vi "Read_DR_DATA.vi"(10 "文件路径":path caption="文件路径 （空时为对话框）") -> (0 "标尺号":i32[](array[numeric]), 1 "时间步长":dbl, 2 "P2数据":dbl[][](array[numeric]), 3 "通量数据":dbl[][](array[numeric]), 4 "曲线数据":dbl[][](array[numeric]), 5 "读取正确?":bool, 6 "曲线名称":string[](array[string]), 8 "数据采集起止时间":string, 11 "filepath":path caption="数据文件路径和名称")   [LabVIEW 2020]
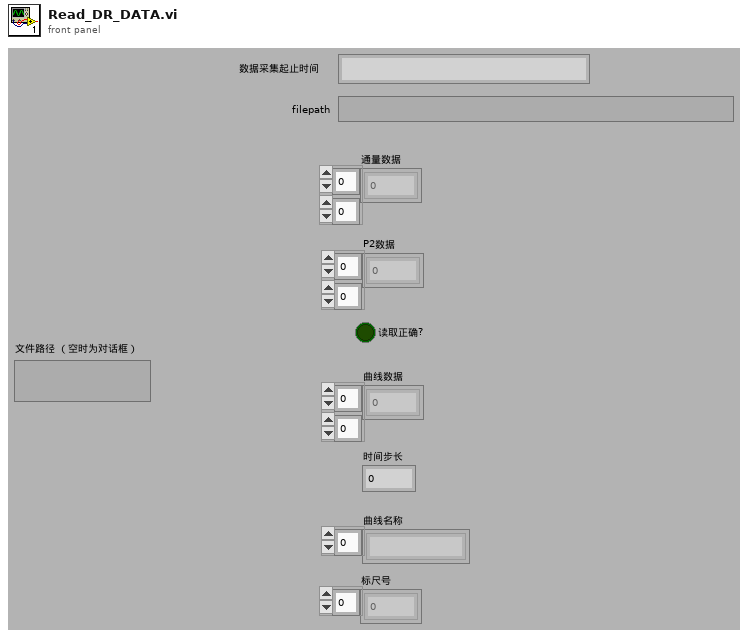
[diagram p1: front panel]
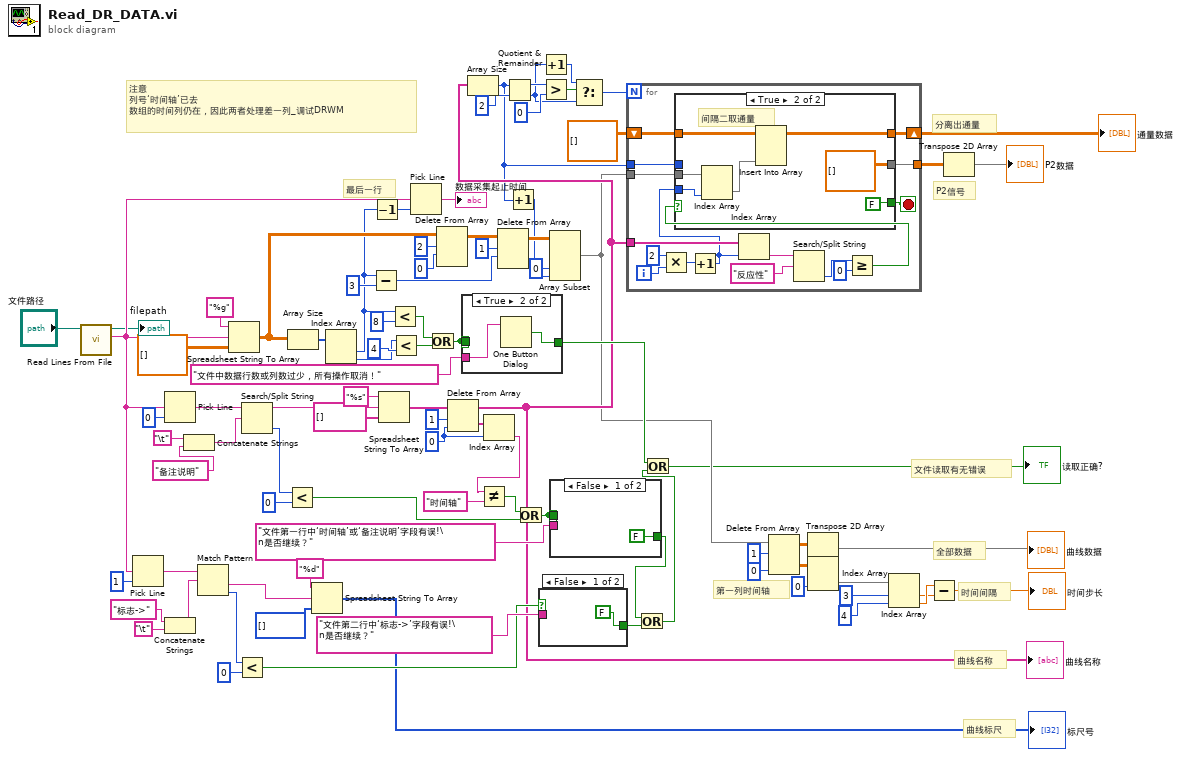
[diagram p0: block diagram]
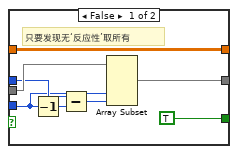
[diagram p2: hidden frame]
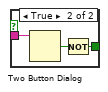
[diagram p3: hidden frame]
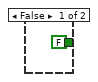
[diagram p4: hidden frame]
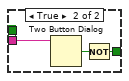
[diagram p5: hidden frame]
diagram:
  w49 = 0 ("索引")
  # "文件读取有无错误"
  # "P2信号"
  # "曲线标尺"
  # "曲线名称"
  # "时间间隔"
  # "全部数据"
  # "分离出通量"
  # "注意\n列号‘时间轴’已去\n数组的时间列仍在，因此两者处理差一列_调试DRWM"
  # "第一列时间轴"
  # "最后一行"
  n1 = call <vilib>:"Read Lines From File.vi"("file path (dialog if empty)"="文件路径") -> ("new file path (Not A Path if cancelled)"=→"filepath":path, "line string"=w39:string)  [unwired: 5 in, 2 out]
  n2 = Pick Line(multi-line string=w39, line index=1 ("行索引")) -> (output string=w66:string)  [unwired: 1 in]
  n3 = Pick Line(multi-line string=w39, line index=0 ("行索引")) -> (output string=w84:string)  [unwired: 1 in]
  n4 = Concatenate Strings("标志->" ("搜索字符串/字符(-)"), "\t") -> (w63:string)
  n5 = Concatenate Strings("\t", "备注说明" ("搜索字符串/字符(-)")) -> (w42:string)
  n6 = Match Pattern(string=w66, regular expression=w63) -> (after substring=w60:string, offset past match=w54:i32)  [unwired: 1 in, 2 out]
  n7 = Spreadsheet String To Array ("电子表格字符串至数组转换")(format string="%g" ("format (%.3f)"), spreadsheet string=w39, array type (2D Dbl)=dbl[][] [] ("type (empty)")) -> (array=w44:dbl[][])  [unwired: 1 in]
  n8 = Less?(x=w54, y=0) -> (x < y?=w53:bool)
  n9 = Search/Split String(string=w84, search string/char (-)=w42) -> (substring before match=w83:string, offset of match=w82:i32)  [unwired: 1 in, 1 out]
  n10 = Less?(x=w82, y=0) -> (x < y?=w79:bool)
  n11 = Array Size(array=w44) -> (size(s)=w90:i32[])
  n12 = Spreadsheet String To Array ("电子表格字符串至数组转换")(format string="%d" ("format (%.3f)"), spreadsheet string=w60, array type (2D Dbl)=i32[] [] ("添加的数组")) -> (array=→"标尺号":i32[])  [unwired: 1 in]
  n13 = Index Array(array=w90) -> (element #1=w12:i32, element #2=w73:i32)  [unwired: 2 in]
  n14 = Subtract(x=w12, y=3) -> (x-y=w38:i32)
  n15 = Decrement(x=w12) -> (x-1=w13:i32)
  n16 = Spreadsheet String To Array ("电子表格字符串至数组转换")(format string="%s" ("format (%.3f)"), spreadsheet string=w83, array type (2D Dbl)=string[] [] ("添加的数组")) -> (array=w52:string[])  [unwired: 1 in]
  n17 = Less?(x=w12, y=8) -> (x < y?=w71:bool)
  n18 = Less?(x=w73, y=4) -> (x < y?=w70:bool)
  n19 = Pick Line(multi-line string=w39, line index=w13) -> (output string=→"数据采集起止时间":string)  [unwired: 1 in]
  n20 = Or(x=w71, y=w70) -> (x .or. y?=w72:bool)
  n21 = Delete From Array(array=w44, length=2 ("长度"), index (row)=0 ("索引")) -> (array with subset deleted=w43:dbl[][])  [unwired: 1 in, 1 out]
  n22 = Delete From Array(array=w52, length=1 ("长度"), index=w49) -> (deleted portion=w50:string[], array with subset deleted=w32:string[])
  "曲线名称" <- w32
  n23 = case shown="True" w72 {
    tunnel: w72 -> [_ _]
    tunnel: [FALSE w92] -> w68
    tunnel: "文件中数据行数或列数过少，所有操作取消！" ("y") -> [_ w93]
    frame False {
    }
    frame True {
      n24 = One Button Dialog(message=w93) -> (true=w92:bool)  [unwired: 1 in]
    }
  }
  n25 = Array Size(array=w32) -> (size(s)=w22:i32)
  n26 = Index Array(array=w50, index=w49) -> (element=w48:string)
  n27 = Not Equal?(x=w48, y="时间轴") -> (x != y?=w78:bool)
  n28 = Delete From Array(array=w43, length=1 ("长度"), index (row)=w38) -> (array with subset deleted=w26:dbl[][])  [unwired: 1 in, 1 out]
  n29 = Quotient & Remainder ("商与余数")(x=w22, y=2) -> (x-y*floor(x/y)=w7:i32, floor(x/y)=w4:i32)
  n30 = Increment(x=w22) -> (x+1=w24:i32)
  n31 = Or(x=w78, y=w79) -> (x .or. y?=w77:bool)
  n32 = case shown="False" w53 {
    tunnel: "文件第二行中‘标志->’字段有误!\n是否继续？" ("y") -> [_ w97]
    tunnel: [FALSE w95] -> w58
    frame False {
    }
    frame True {
      n33 = Two Button Dialog(message=w97) -> (T button?=w96:bool)  [unwired: 2 in]
      n34 = Not(x=w96) -> (.not. x?=w95:bool)
    }
  }
  n35 = Increment(x=w4) -> (x+1=w6:i32)
  n36 = Greater?(x=w7, y=0) -> (0:w8:bool)
  n37 = Array Subset ("数组子集")(array=w26, index (col)=0 ("索引"), length (col)=w24) -> (w25:dbl[][])  [unwired: 2 in]
  n38 = case shown="False" w77 {
    tunnel: w77 -> [_ _]
    tunnel: "文件第一行中‘时间轴’或‘备注说明’字段有误!\n是否继续？" ("y") -> [_ w101]
    tunnel: [FALSE w99] -> w57
    frame False {
    }
    frame True {
      n39 = Two Button Dialog(message=w101) -> (T button?=w100:bool)  [unwired: 2 in]
      n40 = Not(x=w100) -> (.not. x?=w99:bool)
    }
  }
  n41 = Select(t=w6, s=w8, f=w4) -> (s? t:f=w5:i32)
  n42 = for {
    N: w5 -> [_]
    tunnel: w25 -> [w110]
    tunnel: w32 -> [w117]
    shift-right: [w108] -> w35
    shift-left: dbl[][] [] ("type (empty)") -> [w109]
    tunnel: w22 -> [w103]
    tunnel: [w102] -> w34
    i -> [w116]
    stop <- w104 stop-if-true
    n43 = Multiply(x=2, y=w116) -> (x*y=w106:i32)
    n44 = Increment(x=w106) -> (x+1=w105:i32)
    n45 = Index Array(array=w117, index=w105) -> (element=w114:string)
    n46 = Search/Split String(string=w114, search string/char (-)="反应性" ("搜索字符串/字符(-)")) -> (offset of match=w112:i32)  [unwired: 1 in, 2 out]
    n47 = Greater Or Equal?(x=w112, y=0) -> (x >= y?=w107:bool)
    n48 = case shown="True" w107 {
      tunnel: w110 -> [w123 w132]
      tunnel: w109 -> [w125 w131]
      tunnel: [w125 w129] -> w108
      tunnel: w105 -> [w118 w128]
      tunnel: [TRUE FALSE] -> w104
      tunnel: w103 -> [w122 _]
      tunnel: [w120 dbl[][] [] ("type (empty)")] -> w102
      frame False {
        # "只要发现无‘反应性’取所有"
        n49 = Decrement(x=w118) -> (x-1=w119:i32)
        n50 = Subtract(x=w122, y=w119) -> (x-y=w121:i32)
        n51 = Array Subset(array=w123, index (col)=w118, length (col)=w121) -> (w120:dbl[][])  [unwired: 2 in]
      }
      frame True {
        # "间隔二取通量"
        n52 = Index Array(array=w132, index (col)=w128) -> (element=w130:dbl[])  [unwired: 1 in]
        n53 = Insert Into Array(array=w131, new element=w130) -> (w129:dbl[][])  [unwired: 2 in]
      }
    }
  }
  "通量数据" <- w35
  n54 = Or(x=w57, y=w58) -> (x .or. y?=w56:bool)
  n55 = Or(x=w68, y=w56) -> (x .or. y?=→"读取正确?":bool)
  n56 = Delete From Array(array=w25, length=1 ("长度"), index (col)=0 ("禁用的索引 (列)")) -> (deleted portion=w21:dbl[][], array with subset deleted=w29:dbl[][])  [unwired: 1 in]
  n57 = Transpose 2D Array(2D array=w29) -> (transposed array=→"曲线数据":dbl[][])
  n58 = Index Array(array=w21, index (col)=0 ("禁用的索引 (列)")) -> (element=w19:dbl[])  [unwired: 1 in]
  n59 = Index Array(array=w19, index #1=3 ("索引"), index #2=4 ("索引")) -> (element #1=w15:dbl, element #2=w16:dbl)
  n60 = Subtract(x=w16, y=w15) -> (x-y=→"时间步长":dbl)
  n61 = Transpose 2D Array(2D array=w34) -> (transposed array=→"P2数据":dbl[][])
